vi "Get Slave Address Field Width.vi"(8 "error in (no error)":errorcluster, 11 "RFFE Command in":refnum<class "RFFE Command.lvclass">) -> (0 "error out":errorcluster, 2 "Slave Address Field Width":i32, 3 "RFFE Command out":refnum<class "RFFE Command.lvclass">)   [LabVIEW 2018, in "MIPI RFFE API.lvlib" / "RFFE Command.lvclass"]
uses:
  RFFE Command.lvclass
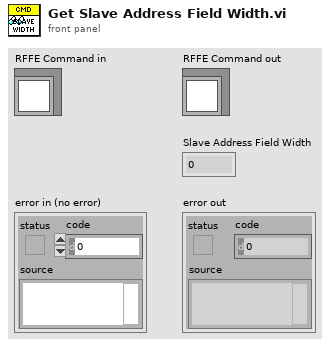
[diagram p1: front panel]
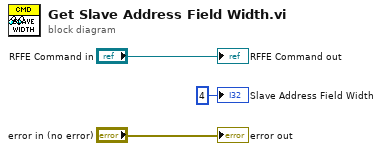
[diagram p0: block diagram]
diagram:
  "error out" <- "error in (no error)"
  "RFFE Command out" <- "RFFE Command in"
  "Slave Address Field Width" <- 4 ("Slave Address Field Width")
